vi "CreatePrivateEvents.vi"(8 "error in (no error)":errorcluster, 11 "SMO.Dictionary":refnum<class "SMO.Dictionary.lvclass">) -> (0 "error out":errorcluster, 3 "SMO.Dictionary out":refnum<class "SMO.Dictionary.lvclass">)   [LabVIEW 2013, in "SMO.Dictionary.lvlib" / "SMO.Dictionary.lvclass"]
doc: "---------------------------------------------------------------\nJKI State Machine Objects™\nhttp://jki.net/state-machine-objects/\nCopyright (C) 2005-2015, JKI <info@jki.net>\nALL RIGHTS RESERVEDJKI State Machine Objects (SMO) 1.0.0.4\nJKI - JKI\nCopyright (c) 2015, JKI"
uses:
  SMO.Dictionary.lvclass
  <vilib>/JKI/JKI SMO/SMO/SMO.lvclass
  Typedefs/PrivateEvents--SMO.Dictionary.KeyValue-Pair.ctl
  Typedefs/PrivateEvents--SMO.Dictionary.Get.ctl
  Typedefs/PrivateEvents--SMO.Dictionary.GetMultipleValues.ctl
  Typedefs/PrivateEvents--SMO.Dictionary.KeyValue-Pair Array.ctl
  SMO.Dictionary.lvclass/SMO.Dictionary.ctl
panel:
  # "For instructions on how to use the JKI State Machine Objects, examples and video tutorials, visit:\nhttp://jki.net/state-machine-objects/\n\nJKI State Machine Objects™\nhttp://jki.net/state-machine-objects/\nCopyright (C) 2005-2015, JKI <info@jki.net>\nALL RIGHTS RESERVED"
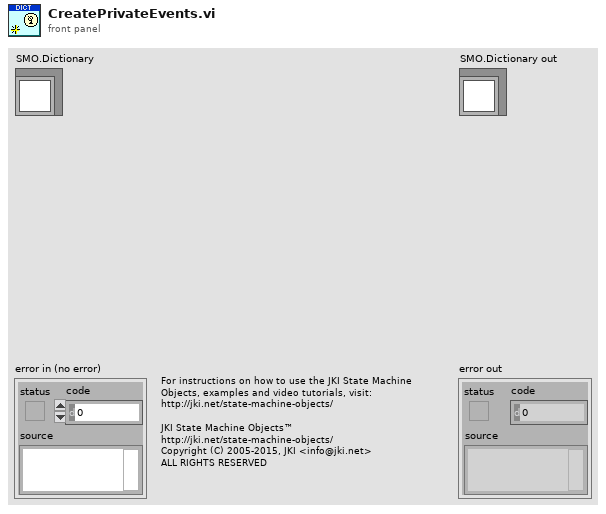
[diagram p1: front panel]
types:
  T1 = typedef "SMO.Dictionary.lvlib/SMO.Dictionary.lvclass/PrivateEvents--SMO.Dictionary.KeyValue-Pair.ctl" = cluster{"Key":string, "Value":variant}
  T2 = typedef "SMO.Dictionary.lvlib/SMO.Dictionary.lvclass/PrivateEvents--SMO.Dictionary.GetMultipleValues.ctl" = cluster{"Keys":string[], "response":refnum<notifier>}
  T3 = typedef "SMO.Dictionary.lvlib/SMO.Dictionary.lvclass/PrivateEvents--SMO.Dictionary.Get.ctl" = cluster{"Key":string, "response":refnum<notifier>}
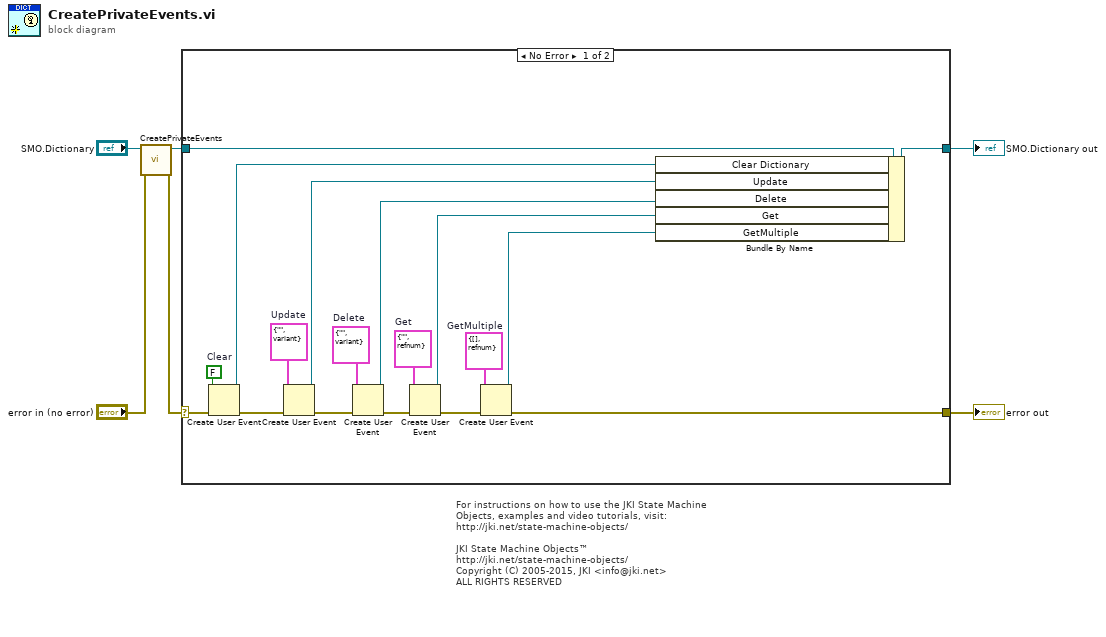
[diagram p0: block diagram]
diagram:
  # "For instructions on how to use the JKI State Machine Objects, examples and video tutorials, visit:\nhttp://jki.net/state-machine-objects/\n\nJKI State Machine Objects™\nhttp://jki.net/state-machine-objects/\nCopyright (C) 2005-2015, JKI <info@jki.net>\nALL RIGHTS RESERVED"
  n1 = call-parent "CreatePrivateEvents.vi"("error in (no error)"="error in (no error)", "SMO"="SMO.Dictionary") -> ("error out"=w1:errorcluster, "SMO out"=w3:refnum<class "SMO.Dictionary.lvclass">)  [unwired: 8 in]
  n2 = case shown="No Error" w1 {
    selector: w1 -> [w23 w26]
    tunnel: [w10 w26] -> w5
    tunnel: [w22 w25] -> w6
    tunnel: w3 -> [w24 w25]
    frame No Error {
      w7 = T1 {"Key"="", "Value"=variant}  # Update
      w9 = T2 {"Keys"=[], "response"=refnum}  # GetMultiple
      w12 = T3 {"Key"="", "response"=refnum}  # Get
      w15 = T1 {"Key"="", "Value"=variant}  # Delete
      w20 = FALSE  # Clear
      n3 = Create User Event(user event datatype=w20, error in=w23) -> (user event=w19:refnum<user-event>, error out=w21:errorcluster)
      n4 = Create User Event(user event datatype=w7, error in=w21) -> (user event=w18:refnum<user-event>, error out=w17:errorcluster)
      n5 = Create User Event(user event datatype=w15, error in=w17) -> (user event=w16:refnum<user-event>, error out=w14:errorcluster)
      n6 = Create User Event(user event datatype=w12, error in=w14) -> (user event=w13:refnum<user-event>, error out=w11:errorcluster)
      n7 = Create User Event(user event datatype=w9, error in=w11) -> (user event=w8:refnum<user-event>, error out=w10:errorcluster)
      n8 = Bundle By Name(cluster=w24, "Clear Dictionary"=w19, "Update"=w18, "Delete"=w16, "Get"=w13, "GetMultiple"=w8) -> (w22:refnum<class "SMO.Dictionary.lvclass">)
    }
    frame Error {
    }
  }
  "error out" <- w5
  "SMO.Dictionary out" <- w6
